vi "OpenTcpDataConnectionSocket.vi"(6 "timeout ms (25000)":i32=30000, 8 "error in":errorcluster, 10 "ConnInfo":T2, 11 "tcp":T1) -> (0 "error out":errorcluster, 3 "ConnectionId":string)   [LabVIEW 2017]
uses:
  <vilib>/addons/InsightCM/MessageBus/Base/controls/ConnectionInfo.ctl
  <vilib>/addons/InsightCM/MessageBus/TcpApi/controls/TcpMessageReference.ctl
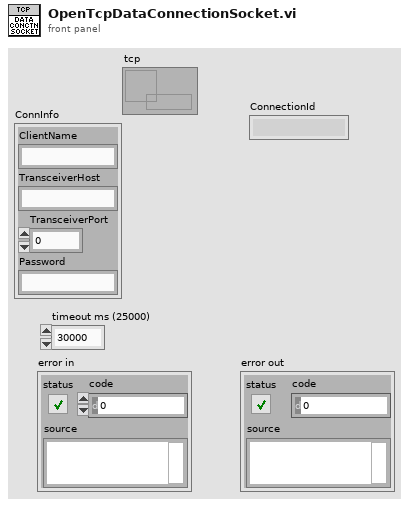
[diagram p1: front panel]
types:
  T1 = typedef "TcpMessageReference.ctl" = refnum<data-value>
  T2 = typedef "ConnectionInfo.ctl" = cluster{"ClientName":string, "TransceiverHost":string, "TransceiverPort":u16, "Password":string}
  T3 = cluster{"AuthDataGUID":string, "ClientName":string}
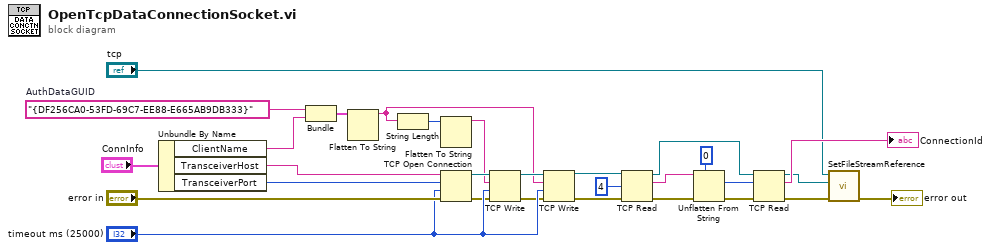
[diagram p0: block diagram]
diagram:
  w17 = "{DF256CA0-53FD-69C7-EE88-E665AB9DB333}"  # AuthDataGUID
  n1 = Unbundle By Name("ConnInfo") -> ("ClientName"=w1:string, "TransceiverHost"=w20:string, "TransceiverPort"=w19:u16)
  n2 = Bundle("AuthDataGUID"=w17, "ClientName"=w1) -> (w9:T3)  [unwired: 1 in]
  n3 = Flatten To String(anything=w9) -> (data string=w12:string)  [unwired: 3 in, 2 out]
  n4 = String Length(string=w12) -> (length=w10:i32)
  n5 = Flatten To String(anything=w10) -> (data string=w11:string)  [unwired: 3 in, 2 out]
  n6 = TCP Open Connection(address=w20, remote port or service name=w19, timeout ms (60000)="timeout ms (25000)", error in (no error)="error in") -> (connection ID=w15:refnum<k5>, error out=w16:errorcluster)  [unwired: 1 in]
  n7 = TCP Write(connection ID=w15, data in=w11, error in (no error)=w16, 9:"timeout ms (25000)") -> (connection ID out=w14:refnum<k5>, error out=w13:errorcluster)  [unwired: 1 out]
  n8 = TCP Write(connection ID=w14, data in=w12, error in (no error)=w13, 9:"timeout ms (25000)") -> (connection ID out=w8:refnum<k5>, error out=w7:errorcluster)  [unwired: 1 out]
  n9 = TCP Read(connection ID=w8, bytes to read=4, error in (no error)=w7) -> (connection ID out=w26:refnum<k5>, data out=w23:string, error out=w27:errorcluster)  [unwired: 2 in]
  n10 = Unflatten From String(type=0, binary string=w23, error in (no error)=w27) -> (value=w25:i32, error out=w28:errorcluster)  [unwired: 2 in, 1 out]
  n11 = TCP Read(connection ID=w26, bytes to read=w25, error in (no error)=w28) -> (connection ID out=w6:refnum<k5>, data out=→"ConnectionId":string, error out=w5:errorcluster)  [unwired: 2 in]
  n12 = call <vilib>:"SetFileStreamReference.vi"("error in (no error)"=w5, "FileStream"=w6, "connection ID out"="tcp") -> ("error out"=→"error out":errorcluster)  [unwired: 7 in, 1 out]
